vi "G Cluster to Struct PLC Byte Stream.vi"(6 "Byte Length":i32, 8 "error in (no error)":errorcluster, 9 "[Sub-Item Type Descriptor]":T1[](array[typedef]), 10 "Value":variant, 11 "TwinCAT ADS in":refnum<class "TwinCAT ADS.lvclass">) -> (0 "error out":errorcluster, 2 "Byte Stream":u8[](array[numeric]), 3 "TwinCAT ADS out":refnum<class "TwinCAT ADS.lvclass">)   [LabVIEW 2018, in "TwinCAT ADS.lvclass"]
uses:
  TwinCAT ADS.lvclass
  Controls/PLC Sub-Item Type Descriptor.ctl
  Controls/PLC Type.ctl
  Controls/PLC Array Type Descriptor.ctl
  G Object to Standard PLC Byte Stream.vi/ebfc1059-5ad7-41af-9a32-6ba056cec1e2.vi
  G Object to Standard PLC Byte Stream.vi/6e01a951-886b-41b5-8cd1-fdd71fd1a533.vi
  G Object to Standard PLC Byte Stream.vi/09c7a0ef-3209-4624-b801-f77696e71225.vi
  G Object to Standard PLC Byte Stream.vi/d245b078-1949-470f-93ac-23e830eec426.vi
  G Object to Standard PLC Byte Stream.vi/0fd4fbf3-4a18-432c-8f70-6a5c8fef8454.vi
  G Object to Standard PLC Byte Stream.vi/afdb5a5e-237c-4be5-828e-15f510cf6cea.vi
  G Object to Standard PLC Byte Stream.vi/185a6e12-4d7d-4ad7-9936-0525adb2f85e.vi
  G Object to Standard PLC Byte Stream.vi/88229fb8-b58c-494b-bd2b-fea6e0d0ed1b.vi
  G Object to Standard PLC Byte Stream.vi/e57df404-389c-41d0-a67c-37c75754ab31.vi
  G Object to Standard PLC Byte Stream.vi/d0ee652c-9b86-46ed-9065-57d03aa8de3e.vi
  G Object to Standard PLC Byte Stream.vi/886bf0b9-f01c-4a44-b2e2-abccc7b97bfa.vi
  G Object to Standard PLC Byte Stream.vi/35f71df7-fc14-4c4d-983c-cf72c138dc9e.vi
  G Object to Standard PLC Byte Stream.vi/2d2bc992-a9ff-4dd8-b8fe-74c21cb85899.vi
  G Object to Standard PLC Byte Stream.vi/100e4a11-5e4a-45b7-be98-adc9eaebd48d.vi
  G Object to Standard PLC Byte Stream.vi/132946d9-68c7-4ade-a66d-dc369520c644.vi
  <vilib>/Utility/error.llb/Trim Whitespace.vi
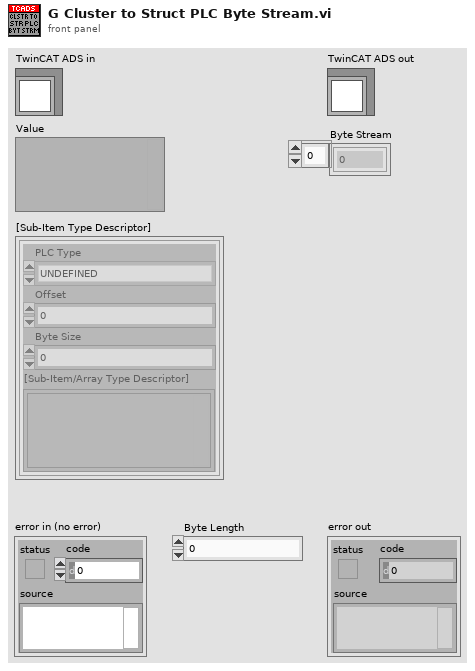
[diagram p1: front panel]
types:
  T1 = typedef "TwinCAT ADS.lvclass/PLC Sub-Item Type Descriptor.ctl" = cluster{"PLC Type":T2, "Offset":i32, "Byte Size":i32, "[Sub-Item/Array Type Descriptor]":variant[]}
  T2 = typedef "TwinCAT ADS.lvclass/PLC Type.ctl" = enum16{"UNDEFINED", "INT", "DINT", "REAL", "LREAL", "SINT", "BYTE", "UINT", "UDINT", "LINT", "ULINT", "STRING", "WSTRING", "BOOL", "TIME", "LTIME", "DATE", "DT", "TOD", "ARRAY", "JAGGED ARRAY", "STRUCT", "FUNCTION BLOCK", "POINTER", "USER DEFINED"}
  T3 = typedef "TwinCAT ADS.lvclass/PLC Array Type Descriptor.ctl" = cluster{"Fundamental PLC Type":T2, "Fundamental Type Byte Size":i32, "Item Count":i32, "Dimension Lengths":i32[], "Sub-Item Type Descriptor":variant}
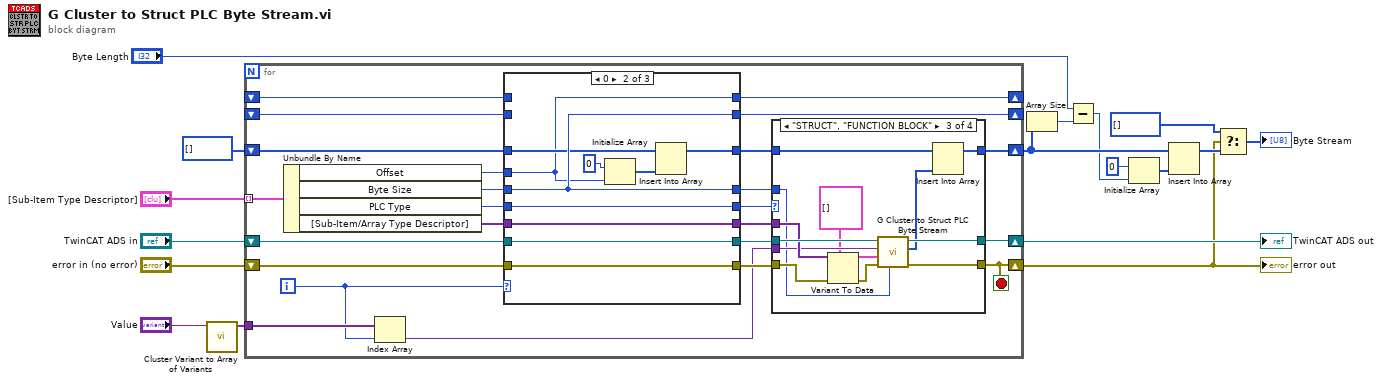
[diagram p0: block diagram]
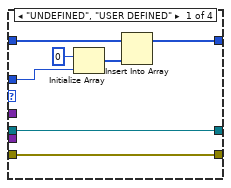
[diagram p2: hidden frame]
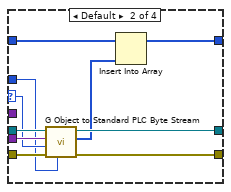
[diagram p3: hidden frame]
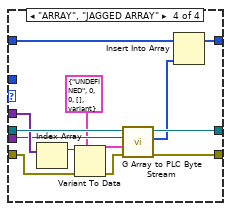
[diagram p4: hidden frame]
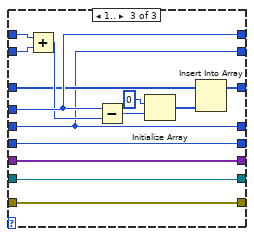
[diagram p6: hidden frame]
diagram:
  n1 = call "Cluster Variant to Array of Variants.vi"("Cluster Variant"="Value") -> ("[Variant]"=w11:variant[])  [unwired: 9 in, 1 out]
  n2 = for {
    shift-right: [w37] -> w8
    shift-left: u8[] [] ("Byte Stream") -> [w29]
    shift-right: [w30] -> w16
    shift-left: "TwinCAT ADS in" -> [w41]
    shift-right: [w33] -> _
    shift-left: _ -> [w31]
    shift-right: [w34] -> _
    shift-left: _ -> [w32]
    tunnel: "[Sub-Item Type Descriptor]" -> [w28] mode=indexing
    tunnel: w11 -> [w21]
    shift-right: [w18] -> w3
    shift-left: "error in (no error)" -> [w25]
    i -> [w20]
    stop <- w18 stop-if-true
    n3 = Unbundle By Name(w28) -> ("Offset"=w27:i32, "Byte Size"=w26:i32, "PLC Type"=w23:T2, "[Sub-Item/Array Type Descriptor]"=w24:variant[])
    n4 = Index Array(array=w21, index=w20) -> (element=w19:variant)
    n5 = case shown="0" w20 {
      tunnel: w25 -> [w89 w100 w114]
      tunnel: w24 -> [w88 w98 w112]
      tunnel: w23 -> [w90 w99 w113]
      tunnel: w27 -> [w87 w92 w111]
      tunnel: w26 -> [w85 w97 w102]
      tunnel: w41 -> [w91 w101 w115]
      tunnel: w29 -> [w86 w95 w105]
      tunnel: [w91 w101 w115] -> w40
      tunnel: [w89 w100 w114] -> w39
      tunnel: [w86 w94 w104] -> w38
      tunnel: [w90 w99 w113] -> w36
      tunnel: [w88 w98 w112] -> w35
      tunnel: [w85 w97 w102] -> w33
      tunnel: [w87 w92 w111] -> w34
      tunnel: w32 -> [_ _ w110]
      tunnel: w31 -> [_ _ w109]
      tunnel: [w85 w97 w102] -> w22
      frame Default {
      }
      frame 0 {
        n6 = Initialize Array(u8 0 ("element"), w92) -> (w93:u8[])
        n7 = Insert Into Array(array=w95, new element=w93) -> (w94:u8[])  [unwired: 1 in]
      }
      frame 1.. {
        n8 = Add(x=w110, y=w109) -> (x+y=w108:i32)
        n9 = Subtract(x=w111, y=w108) -> (x-y=w107:i32)
        n10 = Initialize Array(u8 0 ("element"), w107) -> (w103:u8[])
        n11 = Insert Into Array(array=w105, new element=w103) -> (w104:u8[])  [unwired: 1 in]
      }
    }
    n12 = case shown="\"STRUCT\", \"FUNCTION BLOCK\"" w36 {
      selector: w36 -> [_ w50 _ _]
      tunnel: w40 -> [w48 w58 w71 w84]
      tunnel: w39 -> [w47 w55 w68 w82]
      tunnel: w38 -> [w45 w53 w62 w74]
      tunnel: [w44 w52 w60 w73] -> w37
      tunnel: [w48 w56 w70 w75] -> w30
      tunnel: [w47 w57 w69 w76] -> w18
      tunnel: w35 -> [_ _ w67 w83]
      tunnel: w22 -> [w42 w49 w59 _]
      tunnel: w19 -> [_ w54 w64 w80]
      frame "UNDEFINED", "USER DEFINED" {
        n13 = Initialize Array(u8 0 ("element"), w42) -> (w46:u8[])
        n14 = Insert Into Array(array=w45, new element=w46) -> (w44:u8[])  [unwired: 1 in]
      }
      frame Default {
        n15 = call "G Object to Standard PLC Byte Stream.vi"("Byte Length"=w49, "error in (no error)"=w55, "PLC Type"=w50, "Value"=w54, "TwinCAT ADS in"=w58) -> ("error out"=w57:errorcluster, "Byte Stream"=w51:u8[], "TwinCAT ADS out"=w56:refnum<class "TwinCAT ADS.lvclass">)  [unwired: 4 in]
        n16 = Insert Into Array(array=w53, new element=w51) -> (w52:u8[])  [unwired: 1 in]
      }
      frame "STRUCT", "FUNCTION BLOCK" {
        n17 = Variant To Data(error in=w68, type=T1[] [] ("[Sub-Item Type Information]"), Variant=w67) -> (data=w65:T1[], error out=w66:errorcluster)
        n18 = call "G Cluster to Struct PLC Byte Stream.vi"("Byte Length"=w59, "error in (no error)"=w66, "[Sub-Item Type Descriptor]"=w65, "Value"=w64, "TwinCAT ADS in"=w71) -> ("error out"=w69:errorcluster, "Byte Stream"=w61:u8[], "TwinCAT ADS out"=w70:refnum<class "TwinCAT ADS.lvclass">)  [unwired: 4 in]
        n19 = Insert Into Array(array=w62, new element=w61) -> (w60:u8[])  [unwired: 1 in]
      }
      frame "ARRAY", "JAGGED ARRAY" {
        n20 = Index Array(array=w83) -> (element=w81:variant)  [unwired: 1 in]
        n21 = Variant To Data(error in=w82, type=T3 {"Fundamental PLC Type"=enum."UNDEFINED", "Fundamental Type Byte Size"=0, "Item Count"=0, "Dimension Lengths"=[], "Sub-Item Type Descriptor"=variant} ("Array Information"), Variant=w81) -> (data=w77:T3, error out=w78:errorcluster)
        n22 = call "G Array to PLC Byte Stream.vi"("error in (no error)"=w78, "Array Information"=w77, "Value"=w80, "TwinCAT ADS in"=w84) -> ("error out"=w76:errorcluster, "Byte Stream"=w72:u8[], "TwinCAT ADS out"=w75:refnum<class "TwinCAT ADS.lvclass">)  [unwired: 5 in]
        n23 = Insert Into Array(array=w74, new element=w72) -> (w73:u8[])  [unwired: 1 in]
      }
    }
  }
  "error out" <- w3
  "TwinCAT ADS out" <- w16
  n24 = Array Size(array=w8) -> (size(s)=w7:i32)
  n25 = Subtract(x="Byte Length", y=w7) -> (x-y=w5:i32)
  n26 = Initialize Array(u8 0 ("element"), w5) -> (w9:u8[])
  n27 = Insert Into Array(array=w8, new element=w9) -> (w4:u8[])  [unwired: 1 in]
  n28 = Select(t=u8[] [] ("Byte Stream"), s=w3, f=w4) -> (s? t:f=→"Byte Stream":u8[])
